vi "Adding Two Integer Numbers.vi"() -> ()   [LabVIEW 2012]
panel:
  out "Integer Result":i16
  in  "Integer Two":i16
  in  "Integer One":i16
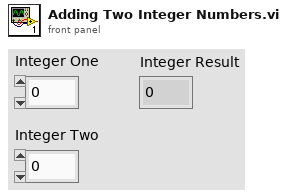
[diagram p1: front panel]
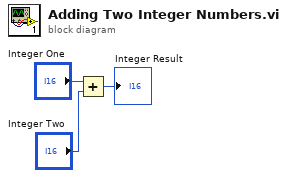
[diagram p0: block diagram]
diagram:
  n1 = Add(x="Integer One", y="Integer Two") -> (x+y=→"Integer Result":i16)
